vi "Parse DB Channel.vi"(0 "XMLBoardConfig in":refnum<k20>, 5 "BoardConfigHandle in":u32, 11 "Error in":errorcluster) -> (4 "XMLBoardConfig out":refnum<k20>, 6 "BoardConfigHandle out":u32, 8 "Array":T1[](array[typedef]) {"speed" items=["OWL429_HIGH_SPEED_CHANNEL", "OWL429_LOW_SPEED_CHANNEL"]; "Labels"."scheduleBuildUnit" items=["Millisecond", "Microsecond"]}, 15 "Error out":errorcluster)   [LabVIEW 2016]
doc: "Parse DB Channel"
uses:
  <userlib>/ARINC-429/Owl429.lvlib
  Ballard Arinc-429 System Explorer.lvlib
  Controls/ARINCParam.ctl
  Controls/AIT_Word.ctl
  Shared/Controls and Global/TransferType.ctl
  Shared/Ballard Arinc-429 Shared.lvlib
  Controls/AIT_Label.ctl
  Controls/Ballard_Channel.ctl
  Controls/Channel Speed.ctl
  Controls/Channel_direction.ctl
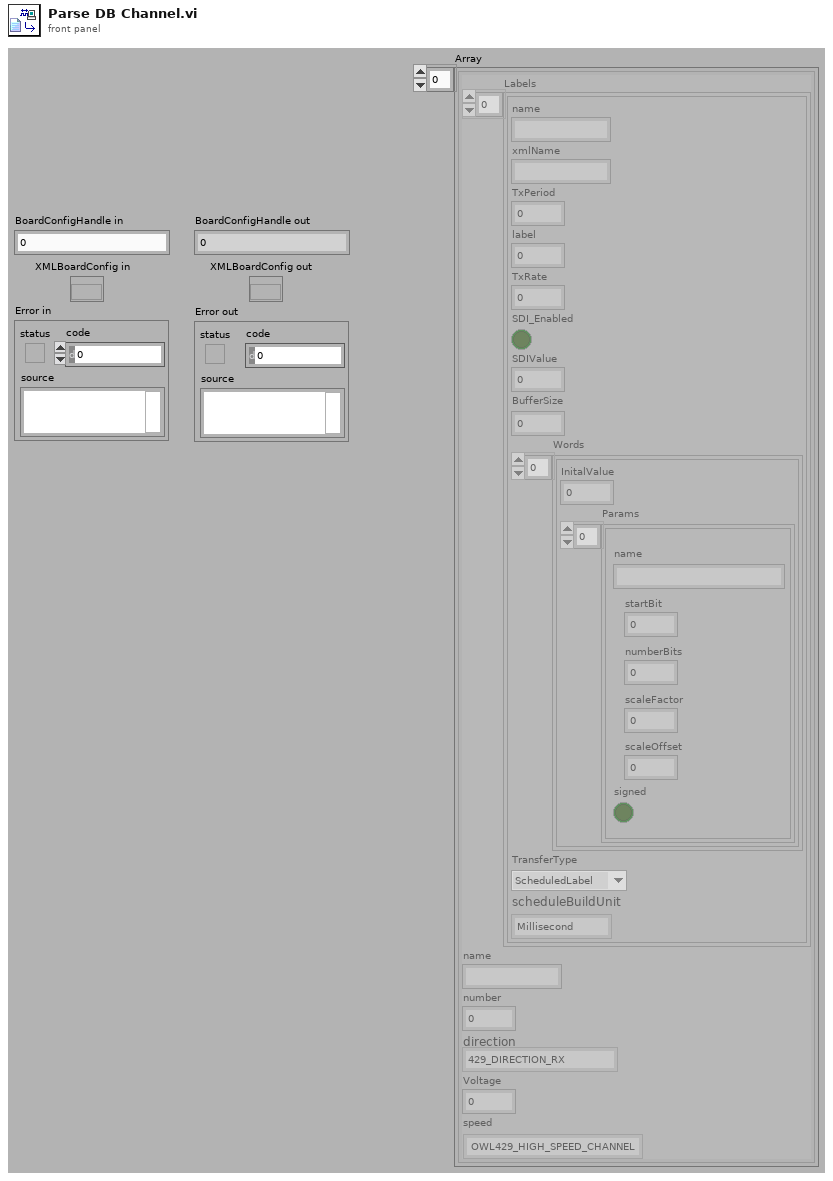
[diagram p1: front panel]
types:
  T1 = typedef "Ballard Arinc-429 System Explorer.lvlib/Ballard_Channel.ctl" = cluster{"Labels":T2[], "name":string, "number":u8, "direction":T6, "Voltage":dbl, "speed":T7}
  T2 = typedef "Ballard Arinc-429 System Explorer.lvlib/AIT_Label.ctl" = cluster{"name":string, "xmlName":string, "TxPeriod":u32, "label":u32, "TxRate":dbl, "SDI_Enabled":bool, "SDIValue":u8, "BufferSize":u32, "Words":T3[], "TransferType":T5, "scheduleBuildUnit":i32}
  T3 = typedef "Ballard Arinc-429 System Explorer.lvlib/AIT_Word.ctl" = cluster{"InitalValue":u32, "Params":T4[]}
  T4 = typedef "Ballard Arinc-429 System Explorer.lvlib/ARINCParam.ctl" = cluster{"name":string, "startBit":i32, "numberBits":i32, "scaleFactor":dbl, "scaleOffset":dbl, "signed":bool}
  T5 = typedef "Ballard Arinc-429 Shared.lvlib/TransferType.ctl" = enum16{"ScheduledLabel", "Acyclic", "Block", "Strobe"}
  T6 = typedef "Channel_direction.ctl" = enum16{"429_DIRECTION_RX", "429_DIRECTION_TX"}
  T7 = typedef "Channel Speed.ctl" = i32
  T8 = enum16{"OWL429_DIRECTION_RX", "OWL429_DIRECTION_TX"}
  T9 = typedef "Owl429.lvlib/Owl429ChannelSpeed.ctl" = i32
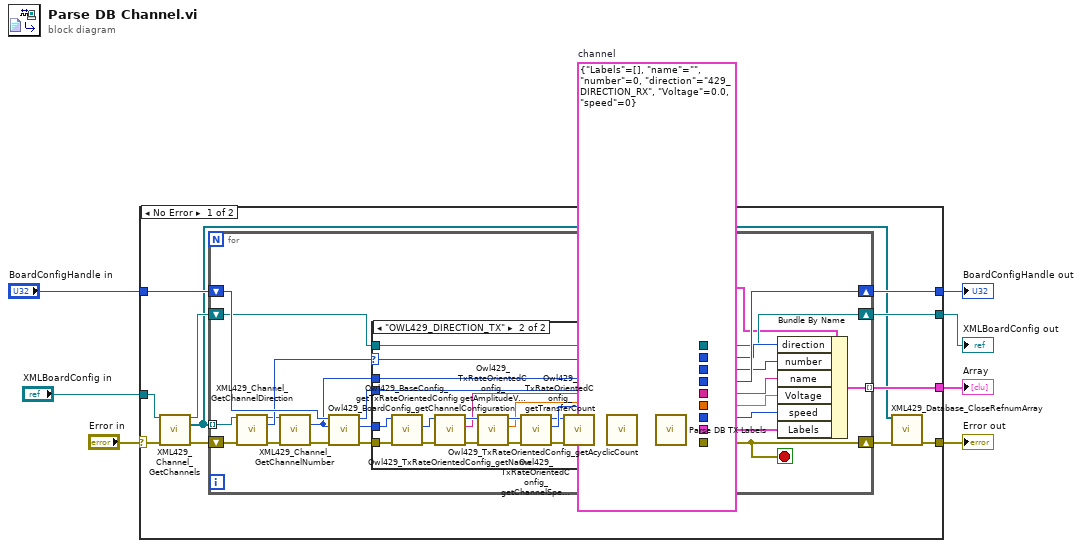
[diagram p0: block diagram]
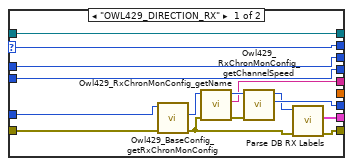
[diagram p2: hidden frame]
diagram:
  n1 = case shown="No Error" "Error in" {
    selector: "Error in" -> [w11 w84]
    tunnel: "BoardConfigHandle in" -> [w18 w83]
    tunnel: [w8 w84] -> w6
    tunnel: [w17 _] -> w1
    tunnel: [w16 w83] -> w5
    tunnel: "XMLBoardConfig in" -> [w12 w82]
    tunnel: [w15 w82] -> w2
    frame No Error {
      n2 = call "XML429_Channel_GetChannels.vi"("BoardConfig in"=w12, "Error in"=w11) -> ("BoardConfig out"=w14:refnum<k20>, "Channels"=w9:refnum<k20>[], "Error out"=w13:errorcluster)  [unwired: 11 in]
      n3 = for {
        shift-right: [w27] -> w10
        shift-left: w13 -> [w24]
        tunnel: [w30] -> w17 mode=indexing
        shift-right: [w41] -> w16
        shift-left: w18 -> [w33]
        tunnel: w9 -> [w25] mode=indexing
        shift-right: [w29] -> w15
        shift-left: w14 -> [w28]
        stop <- w27 stop-if-true
        w19 = T1 {"Labels"=[], "name"="", "number"=0, "direction"=enum."429_DIRECTION_RX", "Voltage"=0.0, "speed"=0}  # channel
        n4 = call "XML429_Channel_GetChannelDirection.vi"("Channel in"=w25, "Error in"=w24) -> ("Channel out"=w23:refnum<k20>, "ChannelDirection"=w26:T8, "Error out"=w22:errorcluster)  [unwired: 11 in]
        n5 = call "XML429_Channel_GetChannelNumber.vi"("Channel in"=w23, "Error in"=w22) -> ("ChannelNumber"=w20:u8, "Error out"=w21:errorcluster)  [unwired: 11 in, 1 out]
        n6 = call <userlib>:"Owl429_BoardConfig_getChannelConfiguration.vi"("error in (no error)"=w21, "channel number"=w20, "board config handle"=w33) -> ("error out"=w40:errorcluster, "base config handle"=w39:u64, "board config handle out"=w36:u64)  [unwired: 6 in]
        n7 = case shown="\"OWL429_DIRECTION_TX\"" w26 {
          selector: w26 -> [w50 w65]
          tunnel: w40 -> [w56 w78]
          tunnel: w39 -> [w55 w77]
          tunnel: [w43 w61] -> w27
          tunnel: [w42 w60] -> w38
          tunnel: [w48 w79] -> w37
          tunnel: [w47 w68] -> w35
          tunnel: [w51 w67] -> w41
          tunnel: w36 -> [w51 w67]
          tunnel: [_ w66] -> w34
          tunnel: w20 -> [w49 w64]
          tunnel: [w50 w65] -> w32
          tunnel: [w49 w64] -> w31
          tunnel: [w46 w63] -> w29
          tunnel: w28 -> [w46 w63]
          frame "OWL429_DIRECTION_RX" {
            n8 = call <userlib>:"Owl429_BaseConfig_getRxChronMonConfig.vi"("error in (no error)"=w56, "config variant handle"=w55) -> ("error out"=w45:errorcluster, "rx config handle"=w54:u64)  [unwired: 7 in, 1 out]
            n9 = call <userlib>:"Owl429_RxChronMonConfig_getName.vi"("error in (no error)"=w45, "config handle"=w54) -> ("error out"=w52:errorcluster, "name"=w47:string, "config handle"=w53:u64)  [unwired: 7 in]
            n10 = call <userlib>:"Owl429_RxChronMonConfig_getChannelSpeed.vi"("error in (no error)"=w52, "config handle"=w53) -> ("speed"=w48:T9, "config handle"=w44:u64)  [unwired: 7 in, 1 out]
            n11 = call "Parse DB RX Labels.vi"("error in"=w45, "config handle"=w44) -> ("error out"=w43:errorcluster, "Labels"=w42:T2[])  [unwired: 8 in]
          }
          frame "OWL429_DIRECTION_TX" {
            n12 = call <userlib>:"Owl429_BaseConfig_getTxRateOrientedConfig.vi"("error in (no error)"=w78, "config variant handle"=w77) -> ("error out"=w76:errorcluster, "tx config handle"=w73:u64)  [unwired: 7 in, 1 out]
            n13 = call <userlib>:"Owl429_TxRateOrientedConfig_getName.vi"("error in (no error)"=w76, "tx config handle"=w73) -> ("error out"=w75:errorcluster, "name"=w68:string, "tx config handle"=w74:u64)  [unwired: 7 in]
            n14 = call <userlib>:"Owl429_TxRateOrientedConfig_getAmplitudeVoltage.vi"("error in (no error)"=w75, "config handle"=w74) -> ("error out"=w81:errorcluster, "voltage"=w66:dbl, "config handle"=w80:u64)  [unwired: 7 in]
            n15 = call <userlib>:"Owl429_TxRateOrientedConfig_getChannelSpeed.vi"("error in (no error)"=w81, "config handle"=w80) -> ("error out"=w72:errorcluster, "speed"=w79:T9, "config handle"=w71:u64)  [unwired: 7 in]
            n16 = call <userlib>:"Owl429_TxRateOrientedConfig_getTransferCount.vi"("error in (no error)"=w72, "config handle"=w71) -> ("error out"=w70:errorcluster, "transfer count"=w58:u32, "config handle"=w69:u64)  [unwired: 7 in]
            n17 = call <userlib>:"Owl429_TxRateOrientedConfig_getAcyclicCount.vi"("error in (no error)"=w70, "config handle"=w69) -> ("error out"=w62:errorcluster, "count"=w59:u32, "config handle"=w57:u64)  [unwired: 7 in]
            n18 = call "Parse DB TX Labels.vi"("error in"=w62, "acyclic transfer count"=w59, "scheduled transfer count"=w58, "Channel Config"=w57) -> ("error out"=w61:errorcluster, "Labels"=w60:T2[])  [unwired: 6 in]
          }
        }
        n19 = Bundle By Name(cluster=w19, "direction"=w32, "number"=w31, "name"=w35, "Voltage"=w34, "speed"=w37, "Labels"=w38) -> (w30:T1)
      }
      n20 = call "XML429_Database_CloseRefnumArray.vi"("XMLRefnums"=w9, "Error in"=w10) -> ("Error out"=w8:errorcluster)  [unwired: 13 in]
    }
    frame Error {
    }
  }
  "Error out" <- w6
  "BoardConfigHandle out" <- w5
  "XMLBoardConfig out" <- w2
  "Array" <- w1
